vi "Configure test.vi"(6 "Assert VI Path":path, 7 "Existing Queue Elements":string, 8 "error in (no error)":errorcluster, 11 "FP GT in":refnum<class "FP GT.lvclass">) -> (0 "error out":errorcluster, 3 "FP GT out":refnum<class "FP GT.lvclass">)   [LabVIEW 2018, in "FP GT.lvclass"]
uses:
  FP GT.lvclass
  11cfa323-248f-44bc-bb35-a55c4c5683da.vi
  <vilib>/JDP Science/JSONtext/Find Item.vi
  11cfa323-248f-44bc-bb35-a55c4c5683da.vi/f6f8fe63-a586-43c8-bfb7-472555a50065.vi
  11cfa323-248f-44bc-bb35-a55c4c5683da.vi/4dd4c385-1307-47f6-8ef9-7aaf3168738c.vi
  <vilib>/JDP Science/JSONtext/String Subset.vi
  Test Class String IDs.vi
  <vilib>/JDP Science/JSONtext/Parsing/Parse Full Path or Item Name.vi
  <vilib>/JDP Science/JSONtext/Offset/Find Item Locations by Path.vi
  <vilib>/JDP Science/JSONtext/JSON text to Variant.vi
  <vilib>/JDP Science/JSONtext/Variant to JSON Text.vi
  <vilib>/JDP Science/JSONtext/Set Item.vi
  Floating Point.lvclass
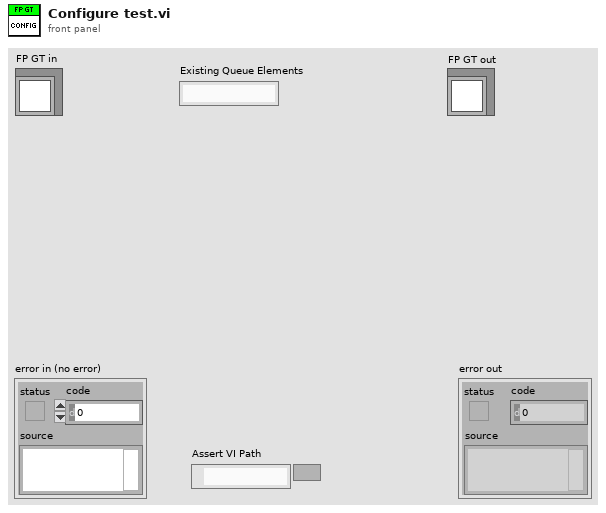
[diagram p1: front panel]
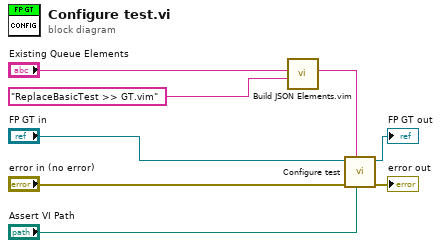
[diagram p0: block diagram]
diagram:
  n1 = call "Build JSON Elements.vim"("Append Element(s)"="ReplaceBasicTest >> GT.vim", "JSON Elements in ({})"="Existing Queue Elements") -> ("JSON Elements out"=w1:string)  [unwired: 9 in]
  n2 = call-parent "Configure test.vi"("Assert VI Path"="Assert VI Path", "Existing Queue Elements"=w1, "error in (no error)"="error in (no error)", "Floating Point in"="FP GT in") -> ("error out"=→"error out":errorcluster, "Floating Point out"=→"FP GT out":refnum<class "FP GT.lvclass">)  [unwired: 6 in]
